vi "Auto_PID_Drive.vi"(5 "Turning_PID_Enable":bool, 6 "dt (s)":dbl=10.0 format="%.3f", 7 "Turning_Setpoint":dbl, 8 "Yaw":dbl=-13.119872265000097, 9 "Turning":dbl, 10 "Power":dbl) -> (2 "Turning":dbl, 3 "Power":dbl)   [LabVIEW 2016]
uses:
  <vilib>/Rock Robotics/Network Tables/NT Read Number.vi
  <vilib>/Rock Robotics/Network Tables/NT Write Number.vi
  <vilib>/addons/control/pid/pid.llb/PID (DBL).vi
  <vilib>/addons/control/pid/NI_PID_pid.lvlib
panel:
  out "Error":dbl
  out "Waveform Chart 2":dbl(graph)
  out "Waveform Chart":cluster{"Turning_Setpoint":dbl, "Yaw":dbl}(graph)={"Turning_Setpoint"=0.0, "Yaw"=-13.119872265000097}
  in  "PID Gains":T1={"proportional gain (Kc)"=0.09, "integral time (Ti, min)"=0.9, "derivative time (Td, min)"=0.001}
  # "1/24/17\nKc=0.015\nTi=5\nTd=0.0005\nTurns slowly, but well"
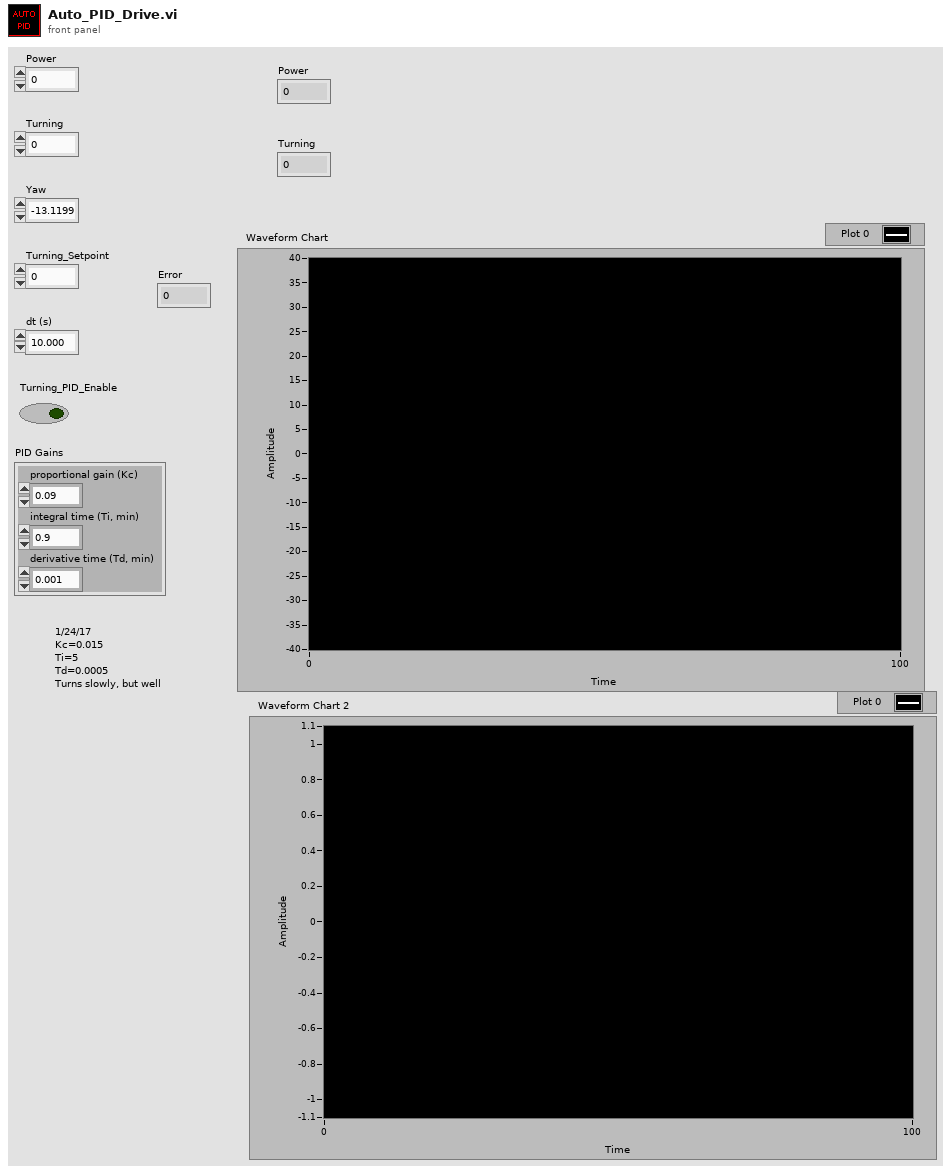
[diagram p1: front panel]
types:
  T1 = cluster{"proportional gain (Kc)":dbl, "integral time (Ti, min)":dbl, "derivative time (Td, min)":dbl}
  T2 = cluster{"Power":dbl, "Yaw":dbl, "Turning_PID_Enable":bool, "Turning":dbl, "Turning_Setpoint":dbl, "PID Gains":cluster{"proportional gain (Kc)":dbl, "integral time (Ti, min)":dbl, "derivative time (Td, min)":dbl}, "dt (s)":dbl}
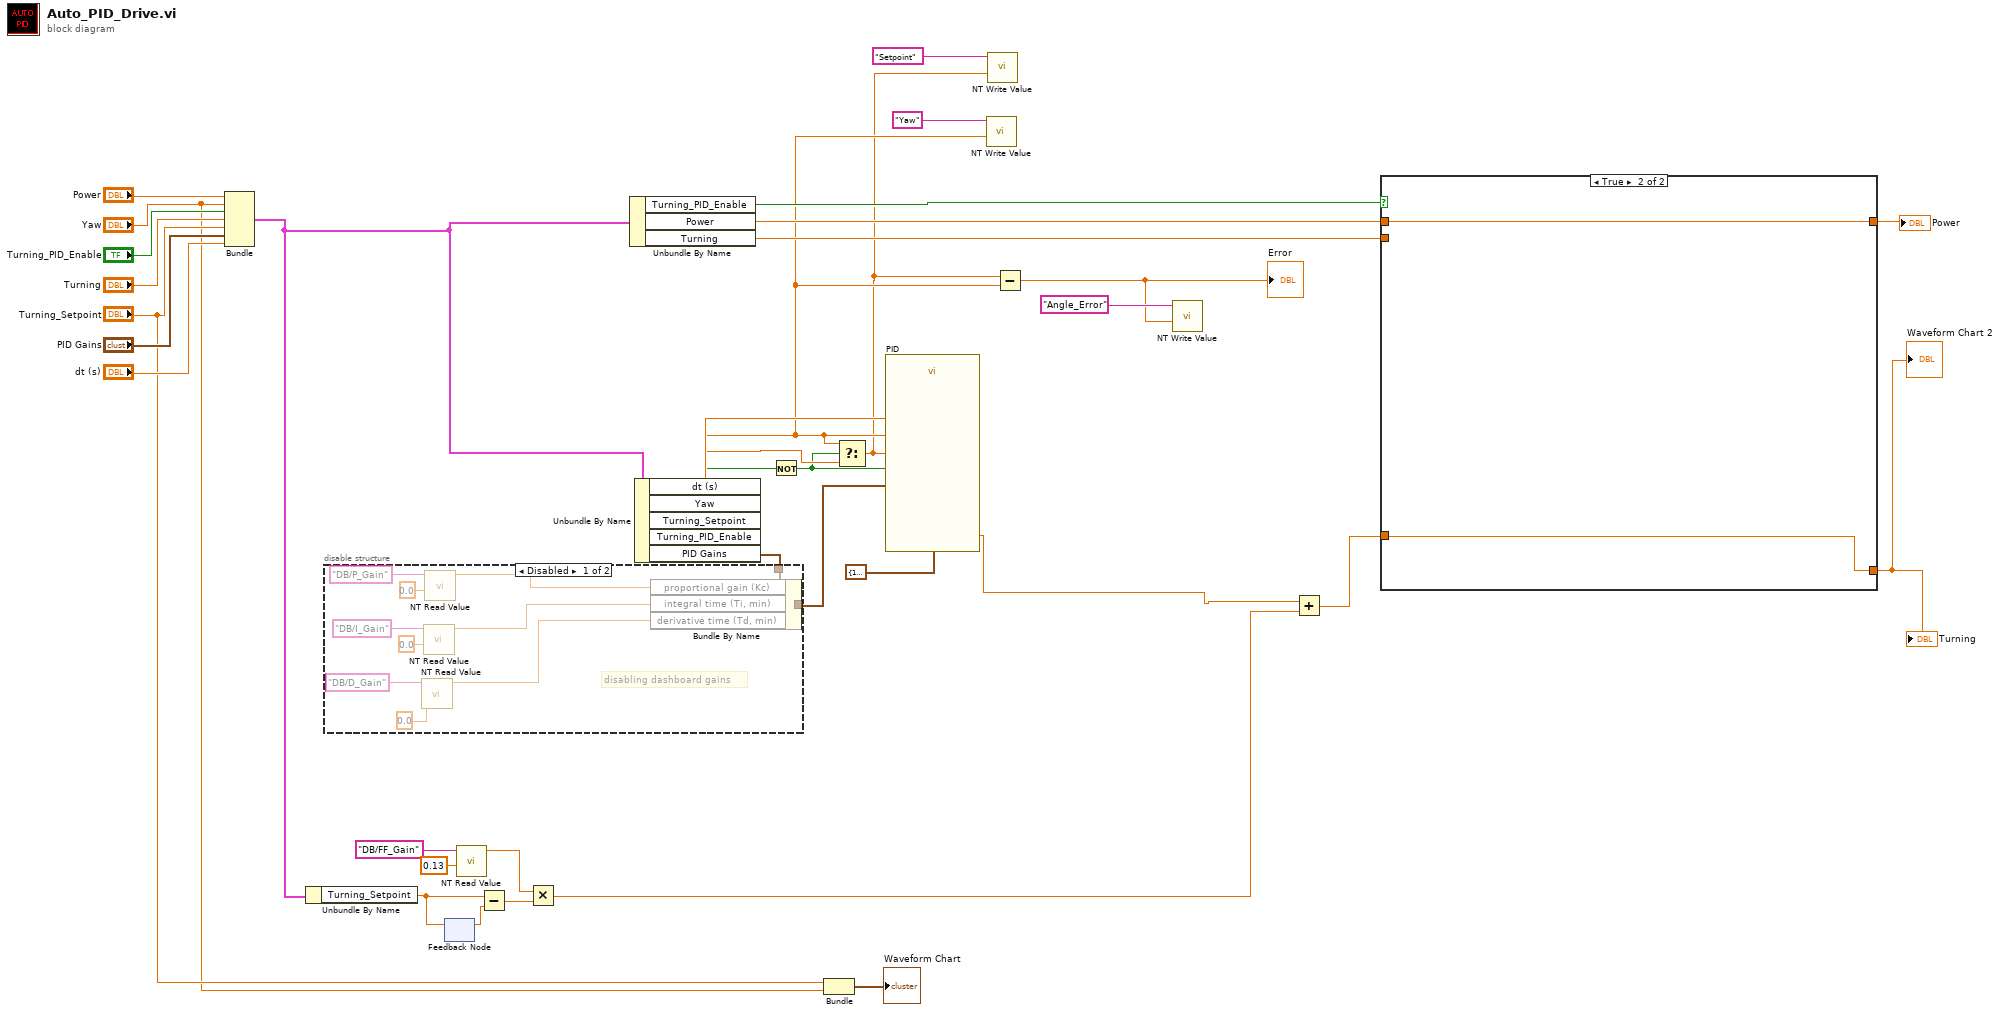
[diagram p0: block diagram]
diagram:
  n1 = Bundle("Power"="Power", "Yaw"="Yaw", "Turning_PID_Enable"="Turning_PID_Enable", "Turning"="Turning", "Turning_Setpoint"="Turning_Setpoint", "PID Gains"="PID Gains", "dt (s)"="dt (s)") -> (w22:T2)  [unwired: 1 in]
  n2 = Unbundle By Name(w22) -> ("Turning_Setpoint"=w25:dbl)
  n3 = feedback-in #1(w25) -> ()
  n4 = feedback #1() -> (w24:dbl)  [unwired: 1 in]
  n5 = call-poly <vilib>:"NT Read Value.vi"("Default Value"=0.13, "Name"="DB/FF_Gain" ("refnum name")) -> ("Numeric"=w10:dbl)  [unwired: 8 in, 1 out]
  n6 = Subtract(x=w25, y=w24) -> (x-y=w23:dbl)
  n7 = Multiply(x=w10, y=w23) -> (x*y=w18:dbl)
  n8 = Unbundle By Name(w22) -> ("Turning_PID_Enable"=w21:bool, "Power"=w26:dbl, "Turning"=w32:dbl)
  n9 = Unbundle By Name(w22) -> ("dt (s)"=w17:dbl, "Yaw"=w5:dbl, "Turning_Setpoint"=w14:dbl, "Turning_PID_Enable"=w16:bool, "PID Gains"=w1:T1)
  n10 = disable-structure shown="Disabled" {
    disable-tunnel: [w46 w48] -> w2
    disable-tunnel: [w37 _] -> _
    disable-tunnel: w1 -> [w37 w48]
    frame Disabled {
      # "disabling dashboard gains"
      n11 = call-poly <vilib>:"NT Read Value.vi"("Default Value"=0.0, "Name"="DB/D_Gain" ("refnum name")) -> ("Numeric"=w39:dbl)  [unwired: 8 in, 1 out]
      n12 = call-poly <vilib>:"NT Read Value.vi"("Default Value"=0.0, "Name"="DB/I_Gain" ("refnum name")) -> ("Numeric"=w40:dbl)  [unwired: 8 in, 1 out]
      n13 = call-poly <vilib>:"NT Read Value.vi"("Default Value"=0.0, "Name"="DB/P_Gain" ("refnum name")) -> ("Numeric"=w41:dbl)  [unwired: 8 in, 1 out]
      n14 = Bundle By Name(cluster=w37, "proportional gain (Kc)"=w41, "integral time (Ti, min)"=w40, "derivative time (Td, min)"=w39) -> (w46:T1)
    }
    frame Enabled {
    }
  }
  n15 = Not(x=w16) -> (.not. x?=w13:bool)
  n16 = Bundle("Turning_Setpoint"="Turning_Setpoint", "Yaw"="Yaw") -> (→"Waveform Chart":cluster{"Turning_Setpoint":dbl, "Yaw":dbl})  [unwired: 1 in]
  n17 = Select(t=w5, s=w13, f=w14) -> (s? t:f=w4:dbl)
  n18 = call-poly <vilib>:"PID.vi"("reinitialize? (F)"=w13, "output range"=cluster{"output high":dbl, "output low":dbl} {"output high"=1.0, "output low"=-1.0}, "dt (s)"=w17, "PID gains"=w2, "process variable"=w5, "setpoint"=w4) -> ("output"=w3:dbl)  [unwired: 4 in, 1 out]
  n19 = call-poly <vilib>:"NT Write Value.vi"("Numeric"=w5, "Name"="Yaw") -> ()  [unwired: 9 in, 1 out]
  n20 = call-poly <vilib>:"NT Write Value.vi"("Numeric"=w4, "Name"="Setpoint") -> ()  [unwired: 9 in, 1 out]
  n21 = Subtract(x=w4, y=w5) -> (x-y=w8:dbl)
  "Error" <- w8
  n22 = call-poly <vilib>:"NT Write Value.vi"("Numeric"=w8, "Name"="Angle_Error") -> ()  [unwired: 9 in, 1 out]
  n23 = Add(x=w3, y=w18) -> (x+y=w15:dbl)
  n24 = case shown="True" w21 {
    tunnel: w26 -> [w50 w52]
    tunnel: w32 -> [w49 _]
    tunnel: [w50 w52] -> w31
    tunnel: [w49 w51] -> w20
    tunnel: w15 -> [_ w51]
    frame False {
    }
    frame True {
    }
  }
  "Power" <- w31
  "Turning" <- w20
  "Waveform Chart 2" <- w20
